vi "Reset Spy.vi"(8 "error in (no error)":errorcluster, 11 "LabSpy":refnum<data-value>) -> (0 "error out":errorcluster, 3 "LabSpy Out":refnum<data-value>)   [LabVIEW 2013, in "LabSpy.lvclass"]
doc: "Reset the Spy call stack."
uses:
  LabSpy.lvclass
  LabSpy.lvclass/LabSpy.ctl
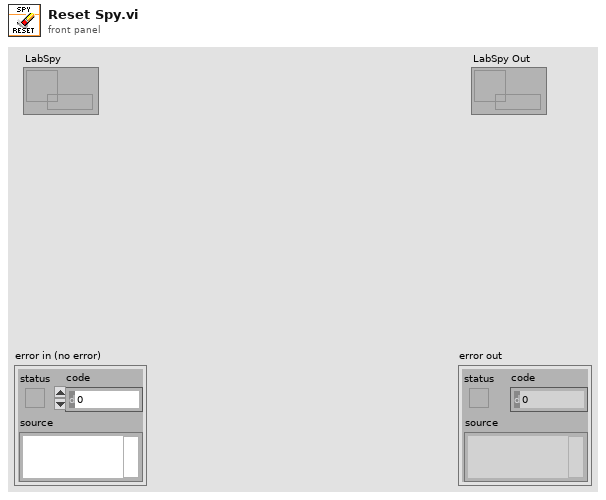
[diagram p1: front panel]
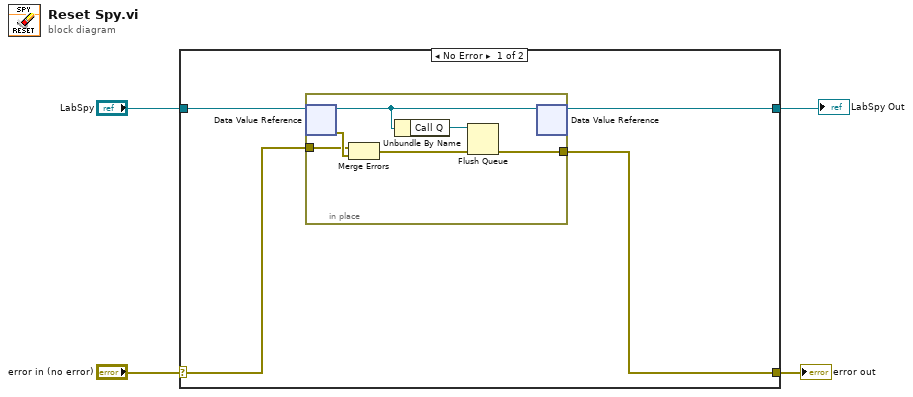
[diagram p0: block diagram]
diagram:
  n1 = case shown="No Error" "error in (no error)" {
    selector: "error in (no error)" -> [w6 w16]
    tunnel: [w5 w16] -> w3
    tunnel: [w7 w15] -> w1
    tunnel: "LabSpy" -> [w8 w15]
    frame No Error {
      n2 = in-place {
        in-place-border: w6 -> [w13]
        in-place-border: [w10] -> w5
        n3 = in-place-dvr #1(w8) -> (w11:refnum<class "LabSpy.lvclass">, w14:errorcluster)
        n4 = Merge Errors(w13, w14) -> (w12:errorcluster)
        n5 = Unbundle By Name(w11) -> ("Call Q"=w9:refnum<queue>)
        n6 = Flush Queue(queue=w9, error in (no error)=w12) -> (error out=w10:errorcluster)  [unwired: 2 out]
        n7 = in-place-dvr #1(w11) -> (w7:refnum<data-value>)  [unwired: 1 out]
      }
    }
    frame Error {
    }
  }
  "error out" <- w3
  "LabSpy Out" <- w1
